vi "Generate String.vi"(8 "error in (no error)":errorcluster, 11 "object in":refnum<class "SetReturnValue.lvclass">) -> (0 "error out":errorcluster, 2 "resulting string":string, 3 "object out":refnum<class "SetReturnValue.lvclass">)   [LabVIEW 2017, in "SetReturnValue.lvclass"]
uses:
  SetReturnValue.lvclass
  SetReturnValue.lvclass/SetReturnValue.ctl
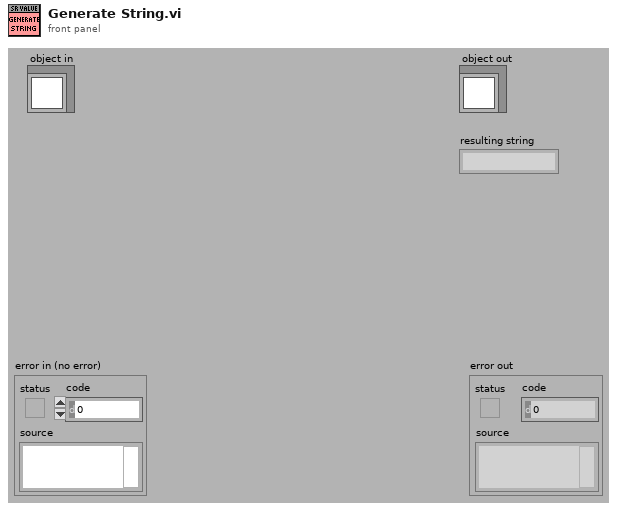
[diagram p1: front panel]
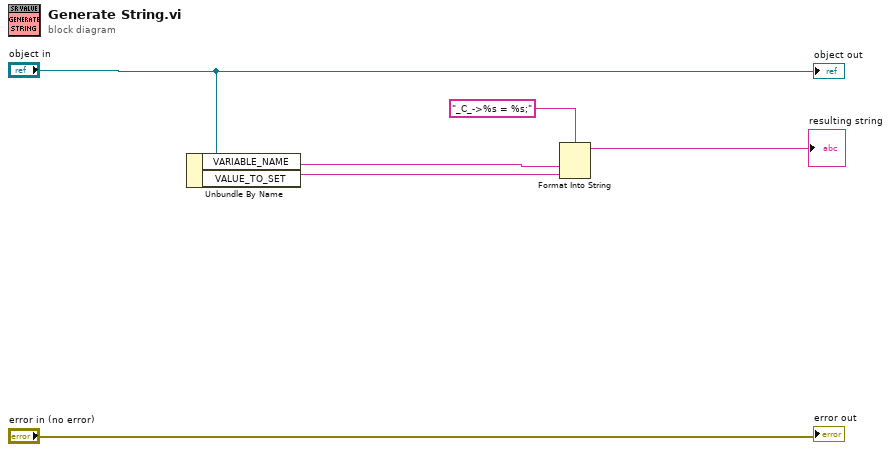
[diagram p0: block diagram]
diagram:
  n1 = Unbundle By Name("object in") -> ("VARIABLE_NAME"=w3:string, "VALUE_TO_SET"=w2:string)
  n2 = Format Into String(format string="_C_->%s = %s;", w3, w2) -> (resulting string=→"resulting string":string)  [unwired: 2 in, 1 out]
  "error out" <- "error in (no error)"
  "object out" <- "object in"
